vi "FWHM (SubVI).vi"(10 "Numeric in":dbl, 11 "horizontalDBL":dbl[](array[numeric])) -> (3 "Numeric out":dbl)   [LabVIEW 2024]
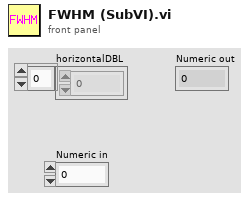
[diagram p1: front panel]
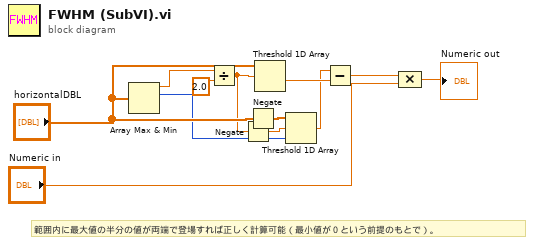
[diagram p0: block diagram]
diagram:
  # "範囲内に最大値の半分の値が両端で登場すれば正しく計算可能（最小値が０という前提のもとで）。"
  n1 = Array Max & Min(array="horizontalDBL") -> (max value=w7:dbl, max index (indices)=w4:i32)  [unwired: 2 out]
  n2 = Divide(x=w7, y=2.0) -> (x/y=w5:dbl)
  n3 = Negate(x=w5) -> (-x=w1:dbl)
  n4 = Negate(x="horizontalDBL") -> (-x=w2:dbl[])
  n5 = Threshold 1D Array(2:w5, 3:"horizontalDBL") -> (0:w9:dbl)  [unwired: 1 in]
  n6 = Threshold 1D Array(1:w4, 2:w1, 3:w2) -> (0:w3:dbl)
  n7 = Subtract(x=w3, y=w9) -> (x-y=w10:dbl)
  n8 = Compound Arithmetic op=MULTIPLY(w10, "Numeric in") -> (→"Numeric out":dbl)
